vi "Set Sciscan Scope Zoom.vi"(8 "error in":errorcluster, 10 "Zoom":dbl=10.0, 11 "GFG Refnum":refnum<vi>) -> (0 "error out":errorcluster, 3 "GFG Refnum Out":refnum<vi>)   [LabVIEW 2012, in "Sciscan Scope Daemon.lvlib"]
uses:
  Sciscan Scope Daemon.lvlib
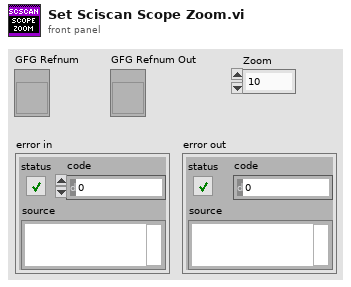
[diagram p1: front panel]
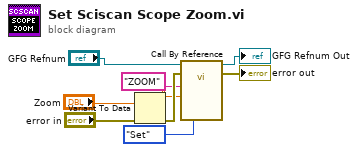
[diagram p0: block diagram]
diagram:
  n1 = Variant To Data(error in="error in", type="Zoom", Variant="Zoom") -> (data=w1:dbl, error out=w9:errorcluster)
  n2 = call-by-ref "?"(reference="GFG Refnum", error in=w9, "Variable Name in"="ZOOM", "Variant in"=w1, "Action"=enum16{"Init", "Set", "Get"}."Set") -> (reference out=→"GFG Refnum Out":refnum<vi>, error out=→"error out":errorcluster)  [unwired: 10 in, 7 out]
